vi "pruebarrayFor.vi"() -> ()   [LabVIEW 2018]
uses:
  <vilib>/Utility/file.llb/Read Delimited Spreadsheet (DBL).vi
panel:
  out "element":dbl
  in  "stop":bool
  out "element 2":dbl
  in  "tiempo":dbl
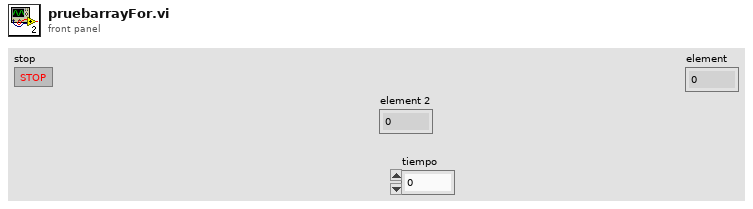
[diagram p1: front panel]
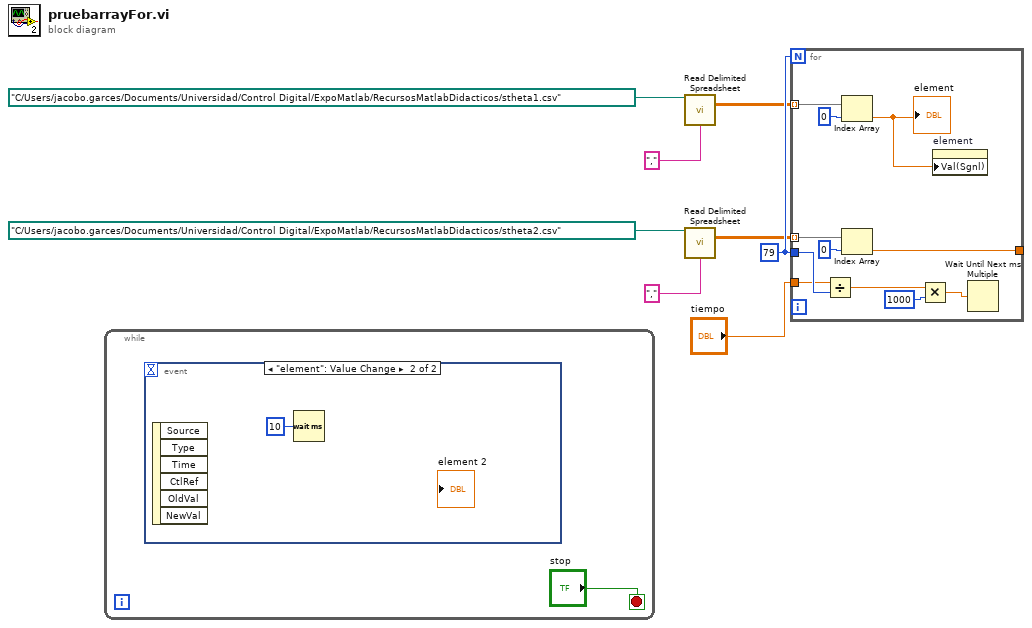
[diagram p0: block diagram]
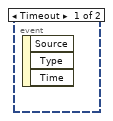
[diagram p2: hidden frame]
diagram:
  w6 = 79
  n1 = while {
    stop <- "stop" stop-if-true
    n2 = event shown="[1] \"element\": Value Change" {
      selector: _ -> [_ _]
      dyn-events: _ -> [_ _]
      timeout: _ -> [_ _]
      event Timeout {
        n3 = event-data() -> ()  [unwired: 1 in, 3 out]
      }
      event "element": Value Change {
        n4 = event-data() -> ()  [unwired: 1 in, 6 out]
        n5 = Wait (ms)(milliseconds to wait=u32 10) -> ()  [unwired: 1 out]
      }
    }
  }
  n6 = call-poly <vilib>:"Read Delimited Spreadsheet.vi"("file path (dialog if empty)"=path "C:/Users/jacobo.garces/Documents/Universidad/Control Digital/ExpoMatlab/RecursosMatlabDidacticos/stheta1.csv", "delimiter (\\t)"="," ("delimiter (\\t)")) -> ("all rows"=w5:dbl[][])  [unwired: 8 in, 5 out]
  n7 = call-poly <vilib>:"Read Delimited Spreadsheet.vi"("file path (dialog if empty)"=path "C:/Users/jacobo.garces/Documents/Universidad/Control Digital/ExpoMatlab/RecursosMatlabDidacticos/stheta2.csv", "delimiter (\\t)"="," ("delimiter (\\t)")) -> ("all rows"=w3:dbl[][])  [unwired: 8 in, 5 out]
  n8 = for {
    N: w6 -> [_]
    tunnel: w6 -> [w19]
    tunnel: w5 -> [w18] mode=indexing
    tunnel: "tiempo" -> [w16]
    tunnel: w3 -> [w14] mode=indexing
    tunnel: [w13] -> _
    n9 = Divide(x=w16, y=w19) -> (x/y=w21:dbl)
    n10 = Index Array(array=w18, index=0) -> (element=w11:dbl)
    "element" <- w11
    n11 = Index Array(array=w14, index=0) -> (element=w13:dbl)
    n12 = Multiply(x=w21, y=1000) -> (x*y=w12:dbl)
    n13 = property on="element" class="DigNum (strict)"("Val(Sgnl)"=w11) -> ()  [unwired: 2 in, 2 out]
    n14 = Wait Until Next ms Multiple(millisecond multiple=w12) -> ()  [unwired: 1 out]
  }
